vi "Circulo.vi"() -> ()   [LabVIEW 2020]
panel:
  out "Gráfico de un circulo":cluster{"X":dbl, "Y":dbl}[](graph)
  # "Diego Jáuregui Ontiveros\nCarlos Uriel Casas Casas\nAlejandro López González"
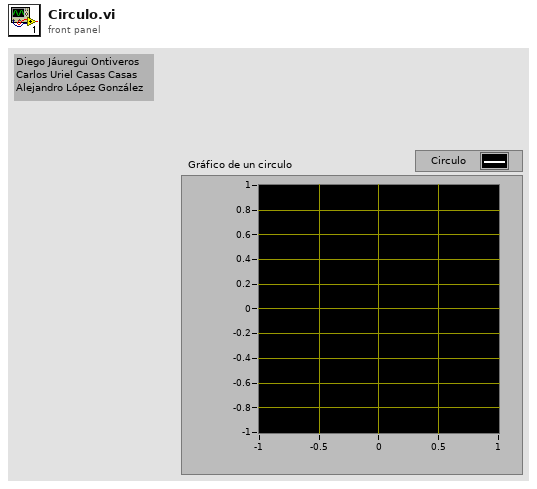
[diagram p1: front panel]
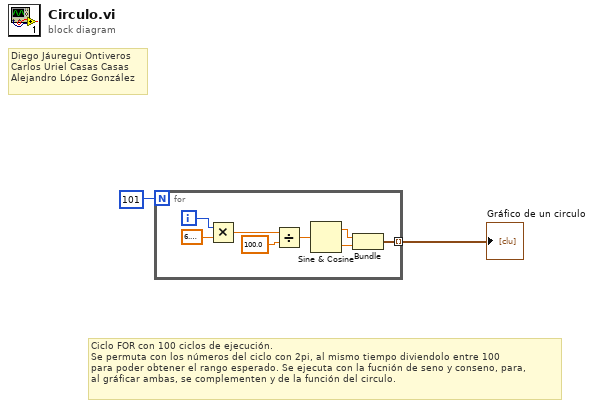
[diagram p0: block diagram]
diagram:
  # "Ciclo FOR con 100 ciclos de ejecución.\nSe permuta con los números del ciclo con 2pi, al mismo tiempo diviendolo entre 100\npara poder obtener el rango esperado. Se ejecuta con la fucnión de seno y conseno, para,\nal gráficar ambas, se complementen y de la función del circulo."
  # "Diego Jáuregui Ontiveros\nCarlos Uriel Casas Casas\nAlejandro López González"
  n1 = for {
    N: 101 -> [_]
    tunnel: [w4] -> w1 mode=indexing
    i -> [w9]
    n2 = Multiply(x=w9, y=6.283185307179586) -> (x*y=w8:dbl)
    n3 = Divide(x=w8, y=100.0) -> (x/y=w6:dbl)
    n4 = Sine & Cosine(0:w6) -> (1:w5:dbl, 2:w3:dbl)
    n5 = Bundle(w5, w3) -> (w4:cluster{dbl, dbl})  [unwired: 1 in]
  }
  "Gráfico de un circulo" <- w1
